vi "CannonProjectileGameFramework-Original.vi"() -> ()   [LabVIEW 2018]
panel:
  out "Distance":dbl
  out "?":cluster{dbl[], dbl[]}(graph)
  out "Score":dbl
  out "Attempt":i32
  out "Wind (mph)":dbl
  out "Target Distance (m)":dbl
  in  "?":bool
  in  "?":bool
  in  "Height (m)":dbl
  in  "Power":dbl
  in  "Angle (deg)":dbl
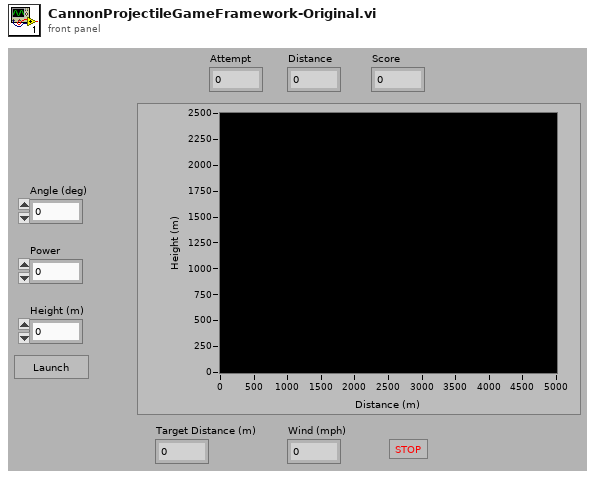
[diagram p1: front panel]
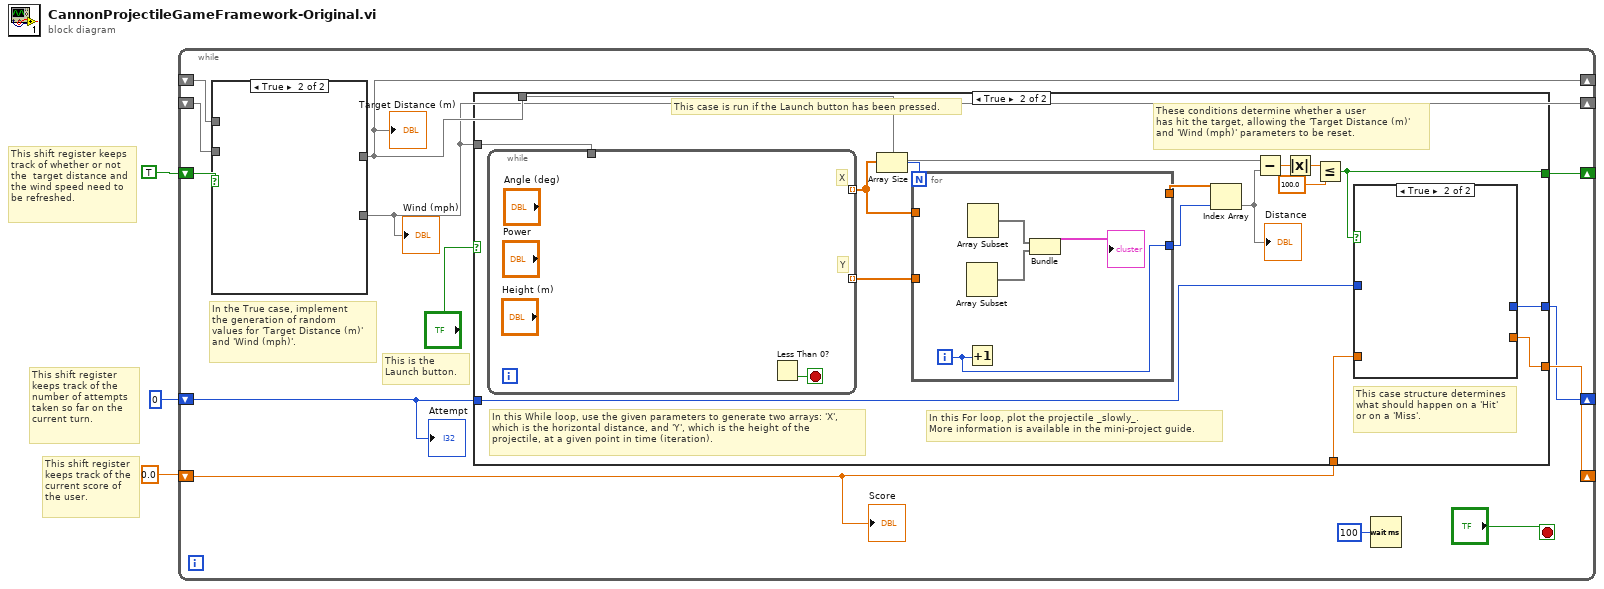
[diagram p0: block diagram]
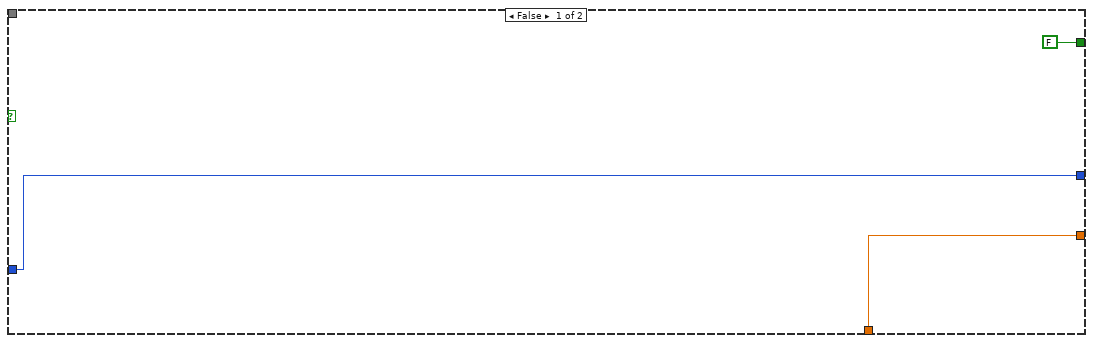
[diagram p3: hidden frame]
diagram:
  # "This shift register keeps\ntrack of whether or not\nthe  target distance and\nthe wind speed need to\nbe refreshed."
  # "This shift register\nkeeps track of the\ncurrent score of\nthe user."
  # "This shift register\nkeeps track of the\nnumber of attempts\ntaken so far on the\ncurrent turn."
  n1 = while {
    shift-right: [w14] -> _
    shift-left: 0.0 -> [w13]
    shift-right: [w12] -> _
    shift-left: 0 -> [w11]
    shift-right: [w9] -> _
    shift-left: TRUE -> [w8]
    shift-right: [w5] -> _
    shift-left: _ -> [w7]
    shift-right: [w4] -> _
    shift-left: _ -> [w6]
    stop <- "?" stop-if-true
    # "This is the Launch button."
    # "In the True case, implement\nthe generation of random\nvalues for 'Target Distance (m)'\nand 'Wind (mph)'."
    n2 = case shown="True" w8 {
      tunnel: [w18 _] -> w5
      tunnel: [w17 _] -> w4
      tunnel: w7 -> [w18 _]
      tunnel: w6 -> [w17 _]
      frame False {
      }
      frame True {
      }
    }
    "Target Distance (m)" <- w5
    "Wind (mph)" <- w4
    n3 = case shown="True" "?" {
      tunnel: w5 -> [_ w36]
      tunnel: w4 -> [_ w37]
      tunnel: [w21 w32] -> w12
      tunnel: w11 -> [w21 w23]
      tunnel: [w20 w25] -> w14
      tunnel: w13 -> [w20 w24]
      tunnel: [FALSE w22] -> w9
      frame False {
      }
      frame True {
        # "These conditions determine whether a user\nhas hit the target, allowing the 'Target Distance (m)'\nand 'Wind (mph)' parameters to be reset."
        # "This case is run if the Launch button has been pressed."
        # "This case structure determines\nwhat should happen on a 'Hit'\nor on a 'Miss'."
        # "In this For loop, plot the projectile _slowly_.\nMore information is available in the mini-project guide."
        # "In this While loop, use the given parameters to generate two arrays: 'X',\nwhich is the horizontal distance, and 'Y', which is the height of the\nprojectile, at a given point in time (iteration)."
        n4 = while {
          tunnel: w37 -> [_]
          tunnel: [_] -> w26 mode=indexing
          tunnel: [_] -> w31 mode=indexing
          stop <- w42 stop-if-true
          # "Y"
          # "X"
          n5 = Less Than 0?() -> (x < 0?=w42:bool)  [unwired: 1 in]
        }
        n6 = Array Size(array=w26) -> (size(s)=w27:i32)
        n7 = for {
          N: w27 -> [_]
          tunnel: w26 -> [_]
          tunnel: w31 -> [_]
          tunnel: [_] -> w30
          tunnel: [w39] -> w29
          i -> [w39]
          n8 = Array Subset() -> (w40:void[])  [unwired: 3 in]
          n9 = Increment(x=w39) -> ()  [unwired: 1 out]
          n10 = Array Subset() -> (w41:void[])  [unwired: 3 in]
          n11 = Bundle(w41, w40) -> (→"?":cluster{void[], void[]})  [unwired: 1 out]
        }
        n12 = Index Array(array=w30, index=w29) -> (element=w28)
        "Distance" <- w28
        n13 = Subtract(x=w36, y=w28) -> (x-y=w35:dbl)
        n14 = Absolute Value(x=w35) -> (abs(x)=w34:dbl)
        n15 = Less Or Equal?(x=w34, y=100.0) -> (x <= y?=w22:bool)
        n16 = case shown="True" w22 {
          tunnel: [_ _] -> w32
          tunnel: w23 -> [_ _]
          tunnel: [_ _] -> w25
          tunnel: w24 -> [_ _]
          frame False {
          }
          frame True {
          }
        }
      }
    }
    n17 = Wait (ms)(milliseconds to wait=u32 100) -> ()  [unwired: 1 out]
    "Score" <- w13
    "Attempt" <- w11
  }
